vi "PSU_CMD_GCFS.vi"(3 "error in":errorcluster, 4 "Connection":bool, 5 "Port":refnum<visa-resource-name>, 6 "output":dbl) -> (0 "error out":errorcluster, 1 "valid?":bool, 2 "Output % duplicate":dbl)   [LabVIEW 2024]
uses:
  cce42e0e-f703-4a6d-af81-a5c4347c74fa.vi
  <vilib>/regexp/Match Regular Expression.xnode
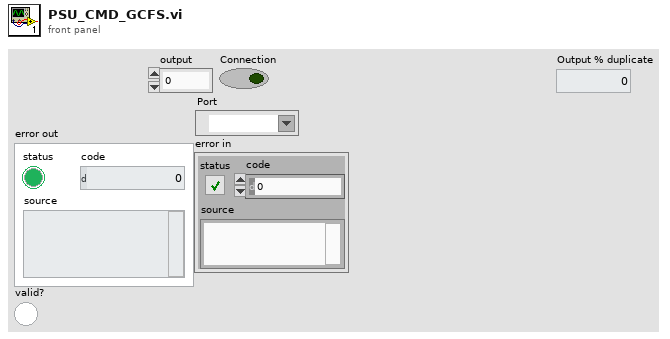
[diagram p1: front panel]
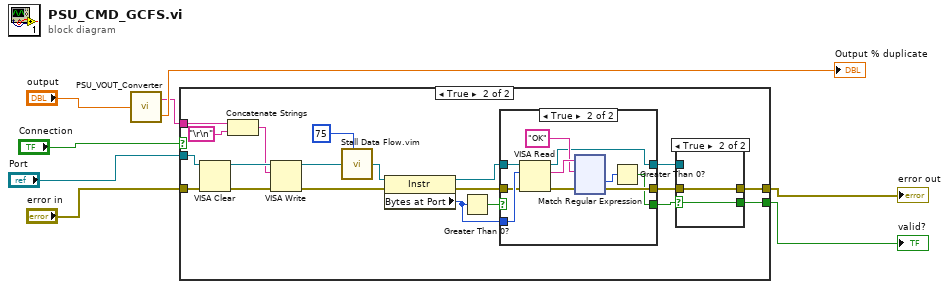
[diagram p0: block diagram]
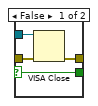
[diagram p3: hidden frame]
diagram:
  n1 = call "PSU_VOUT_Converter.vi"("Output %"="output") -> ("decimal integer string"=w1:string, "Output % duplicate"=→"Output % duplicate":dbl)
  n2 = case shown="True" "Connection" {
    selector: "Connection" -> [w10 _]
    tunnel: "Port" -> [_ w29]
    tunnel: [w9 w23] -> w3
    tunnel: [w10 w22] -> w4
    tunnel: w1 -> [_ w24]
    tunnel: "error in" -> [w9 w20]
    frame False {
    }
    frame True {
      n3 = VISA Clear(VISA resource name=w29, error in (no error)=w20) -> (VISA resource name out=w28:refnum<visa-resource-name>, error out=w27:errorcluster)
      n4 = Concatenate Strings(w24, "\r\n") -> (w21:string)
      n5 = VISA Write(VISA resource name=w28, write buffer=w21, error in (no error)=w27) -> (VISA resource name out=w26:refnum<visa-resource-name>, error out=w25:errorcluster)  [unwired: 1 out]
      n6 = call "Stall Data Flow.vim"("value in"=w26, "milliseconds to wait"=u32 75) -> ("value out"=w19:refnum<visa-resource-name>)  [unwired: 1 out]
      n7 = property class="Instr"(reference=w19, error in=w25) -> (reference out=w16:refnum<visa-resource-name>, error out=w15:errorcluster, "Bytes at Port"=w17:u32)
      n8 = Greater Than 0?(x=w17) -> (x > 0?=w18:bool)
      n9 = case shown="True" w18 {
        selector: w18 -> [w38 _]
        tunnel: w17 -> [_ w49]
        tunnel: w15 -> [w39 w48]
        tunnel: [w39 w43] -> w12
        tunnel: w16 -> [w37 w47]
        tunnel: [w38 w41] -> w13
        tunnel: [w37 w40] -> w11
        frame False {
        }
        frame True {
          n10 = VISA Read(VISA resource name=w47, byte count=w49, error in (no error)=w48) -> (VISA resource name out=w40:refnum<visa-resource-name>, read buffer=w46:string, error out=w45:errorcluster)  [unwired: 1 out]
          n11 = xnode "Match Regular Expression"("input string"=w46, "regular expression"="OK", "error in"=w45) -> ("offset past match"=w42:i32, "error out"=w43:errorcluster)  [unwired: 3 in, 3 out]
          n12 = Greater Than 0?(x=w42) -> (x > 0?=w41:bool)
        }
      }
      n13 = case shown="True" w13 {
        selector: w13 -> [w34 w35]
        tunnel: [w31 w36] -> w23
        tunnel: w12 -> [w32 w36]
        tunnel: [w34 w35] -> w22
        tunnel: w11 -> [w33 _]
        frame False {
          n14 = VISA Close(VISA resource name=w33, error in (no error)=w32) -> (error out=w31:errorcluster)
        }
        frame True {
        }
      }
    }
  }
  "error out" <- w3
  "valid?" <- w4
